vi "UpdateFlag.vi"(7 "LabVIEW Web Service Request":refnum<class "Web Request.lvclass">, 9 "Room":i32, 10 "FlagIn":u32) -> (2 "FlagOut":bool[](array[boolean]))   [LabVIEW 2015]
uses:
  <vilib>/wsapi/Web Request.lvclass
  ActionEnum.ctl
panel:
  # "Use the Web Service Request input terminal to call the VIs on the Web Services palette. Do not remove it from the connector pane unless you don't need access to the palette."
  # "Each additional control wired to the connector pane will be available as an input in the URL. To include an indicator in terminal-mode output (the default setting), it must also be wired to the connector pane."
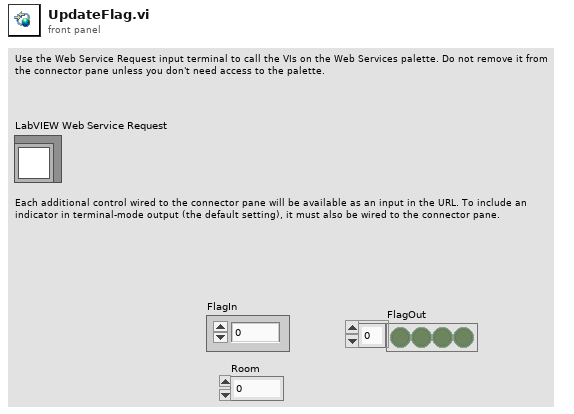
[diagram p1: front panel]
types:
  T1 = typedef "ActionEnum.ctl" = enum16{"Init", "Read", "Write"}
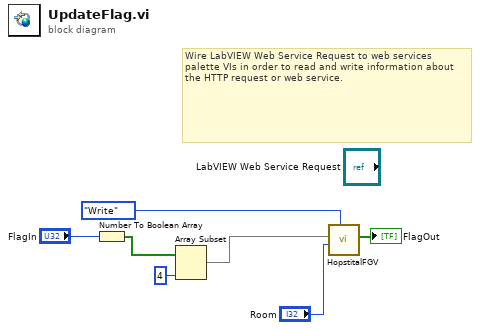
[diagram p0: block diagram]
diagram:
  # "Wire LabVIEW Web Service Request to web services palette VIs in order to read and write information about the HTTP request or web service."
  n1 = Number To Boolean Array(number="FlagIn") -> (Boolean array=w3:bool[])
  n2 = Array Subset(array=w3, length=4) -> (w1:bool[])  [unwired: 1 in]
  n3 = call "HopstitalFGV.vi"(7:ActionEnum."Write", "Room"="Room", "Flag In"=w1) -> ("Flag Out"=→"FlagOut":bool[])  [unwired: 7 in, 1 out]
